vi "图像交错组合与分离2.vi"() -> ()   [LabVIEW 2018]
uses:
  <vilib>/vision/NI_Vision_Development_Module.lvlib
panel:
  out "Image 2":T1(plugin-control)
  out "error out":errorcluster
  out "Image":T1(plugin-control)
  in  "路径":path
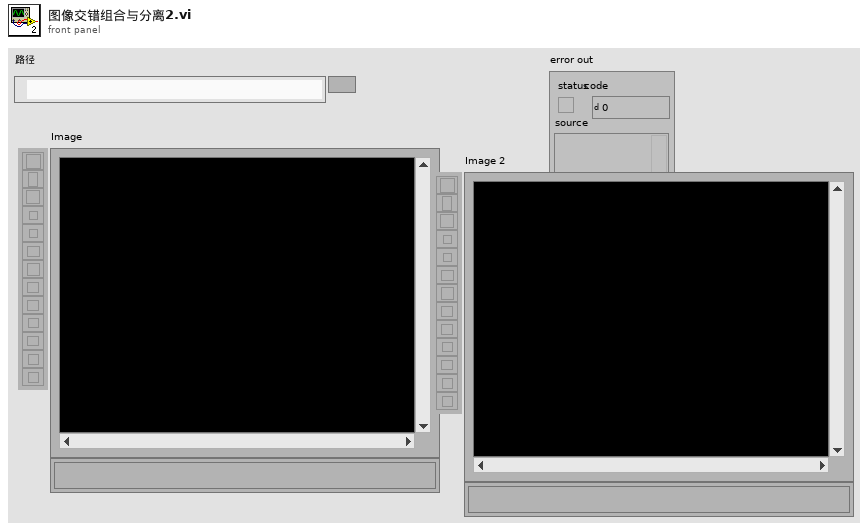
[diagram p1: front panel]
types:
  T1 = typedef "IMAQ Image.ctl" = refnum<image>
  T2 = typedef "Image Type" = u32
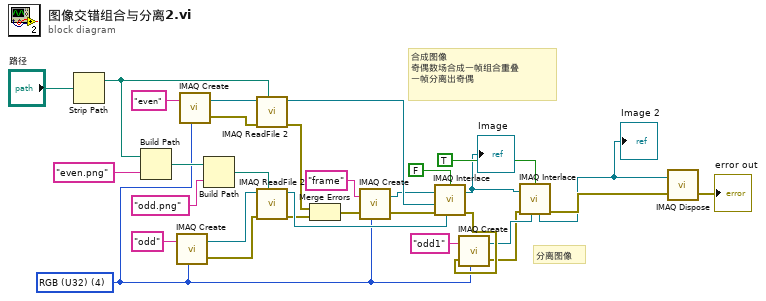
[diagram p0: block diagram]
diagram:
  w2 = T2 4 items=["Grayscale (U8)", "Grayscale (I16)", "Grayscale (SGL)", "Complex (CSG)", "RGB (U32)", "HSL (U32)", "RGB (U64)", "Grayscale (U16)"] ("Image Type")
  # "分离图像"
  # "合成图像\n奇偶数场合成一帧组合重叠\n一帧分离出奇偶"
  n1 = Strip Path(path="路径") -> (stripped path=w21:path)  [unwired: 1 out]
  n2 = Build Path(base path=w21, name or relative path="even.png" ("名称或相对路径")) -> (appended path=w29:path)
  n3 = call "IMAQ Create"("Image Name"="odd", "Image Type"=w2) -> ("New Image"=w25:T1, "error out"=w24:errorcluster)  [unwired: 3 in]
  n4 = call "IMAQ Create"("Image Name"="even", "Image Type"=w2) -> ("New Image"=w22:T1, "error out"=w23:errorcluster)  [unwired: 3 in]
  n5 = Build Path(base path=w29, name or relative path="odd.png" ("名称或相对路径")) -> (appended path=w20:path)
  n6 = call "IMAQ ReadFile 2"("File Path"=w21, "error in (no error)"=w23, "Image"=w22) -> ("error out"=w13:errorcluster, "Image Out"=w19:T1)  [unwired: 4 in, 3 out]
  n7 = call "IMAQ ReadFile 2"("File Path"=w20, "error in (no error)"=w24, "Image"=w25) -> ("error out"=w12:errorcluster, "Image Out"=w18:T1)  [unwired: 4 in, 3 out]
  n8 = Merge Errors(w13, w12) -> (w14:errorcluster)
  n9 = call "IMAQ Create"("Image Name"="frame", "Image Type"=w2, "error in (no error)"=w14) -> ("New Image"=w16:T1, "error out"=w11:errorcluster)  [unwired: 2 in]
  n10 = call "IMAQ Interlace"("error in (no error)"=w11, "Image Even"=w19, "Image Odd"=w18, "Image Frame"=w16, "Interlace/Separate (Interlace)"=FALSE) -> ("error out"=w7:errorcluster, "Image Frame Out"=w5:T1)  [unwired: 2 out]
  "Image" <- w5
  n11 = call "IMAQ Create"("Image Name"="odd1", "Image Type"=w2, "error in (no error)"=w7) -> ("New Image"=w6:T1, "error out"=w4:errorcluster)  [unwired: 2 in]
  n12 = call "IMAQ Interlace"("error in (no error)"=w4, "Image Odd"=w6, "Image Frame"=w5, "Interlace/Separate (Interlace)"=TRUE) -> ("Image Odd Out"=w1:T1, "error out"=w3:errorcluster)  [unwired: 1 in, 2 out]
  "Image 2" <- w1
  n13 = call "IMAQ Dispose"("Image"=w1, "error in (no error)"=w3) -> ("error out"=→"error out":errorcluster)  [unwired: 4 in]
